vi "Project Wizard Caller.vi"() -> ()   [LabVIEW 2021]
panel:
  out "error out":errorcluster
  in  "error in (no error)":errorcluster
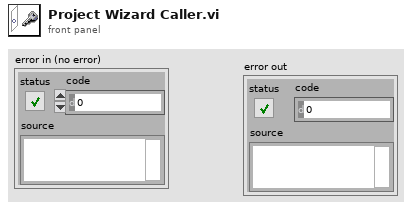
[diagram p1: front panel]
types:
  T1 = enum32{"Invalid", "Standard", "Closed", "Hidden", "Minimized", "Maximized"}
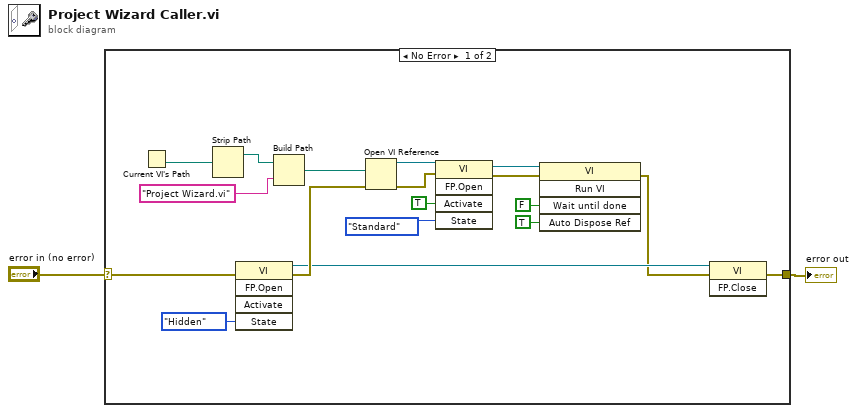
[diagram p0: block diagram]
diagram:
  n1 = case shown="No Error" "error in (no error)" {
    selector: "error in (no error)" -> [w3 w21]
    tunnel: [w4 w21] -> w2
    frame No Error {
      n2 = Current VI's Path() -> (path=w19:path)
      n3 = Strip Path(path=w19) -> (stripped path=w18:path)  [unwired: 1 out]
      n4 = invoke class="VI" method="FP.Open"(error in=w3, "State"=T1."Hidden") -> (reference out=w6:refnum<vi>, error out=w15:errorcluster)  [unwired: 3 in, 3 out]
      n5 = Build Path(base path=w18, name or relative path="Project Wizard.vi") -> (appended path=w16:path)
      n6 = Open VI Reference(vi path=w16, error in (no error)=w15) -> (vi reference=w14:refnum<vi>, error out=w9:errorcluster)  [unwired: 4 in]
      n7 = invoke class="VI" method="FP.Open"(reference=w14, error in=w9, "Activate"=TRUE ("Activate?"), "State"=T1."Standard") -> (reference out=w11:refnum<vi>, error out=w10:errorcluster)  [unwired: 1 in, 3 out]
      n8 = invoke class="VI" method="Run VI"(reference=w11, error in=w10, "Wait until done"=FALSE ("Wait Until Done"), "Auto Dispose Ref"=TRUE ("Auto Dispose Reference")) -> (error out=w5:errorcluster)  [unwired: 1 in, 4 out]
      n9 = invoke class="VI" method="FP.Close"(reference=w6, error in=w5) -> (error out=w4:errorcluster)  [unwired: 1 in, 2 out]
    }
    frame Error {
    }
  }
  "error out" <- w2
